vi "Numerical_Calculation.vi"(11 "Nums":sgl[][](array[numeric]) format="%#.2g") -> (3 "Calculation":sgl[][](array[numeric]) format="%#.2g")   [LabVIEW 2019]
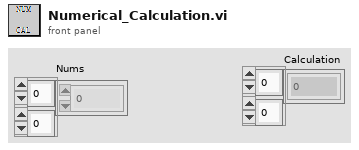
[diagram p1: front panel]
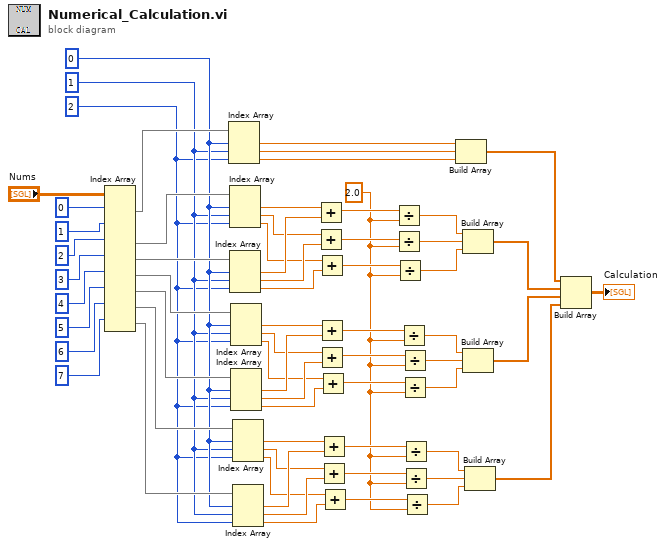
[diagram p0: block diagram]
diagram:
  w18 = sgl 2.0
  w28 = 2
  w29 = 1
  w30 = 0
  n1 = Index Array(array="Nums", index (row) #1=0 ("索引 (行)"), index (row) #2=1 ("索引 (行)"), index (row) #3=2 ("索引 (行)"), index (row) #4=3 ("索引 (行)"), index (row) #5=4 ("索引 (行)"), index (row) #6=5 ("索引 (行)"), index (row) #7=6 ("索引 (行)"), index (row) #8=7 ("索引 (行)")) -> (element #1=w55:sgl[], element #3=w36:sgl[], element #4=w35:sgl[], element #5=w34:sgl[], element #6=w33:sgl[], element #7=w32:sgl[], element #8=w31:sgl[])  [unwired: 8 in, 1 out]
  n2 = Index Array(array=w55, index #1=w30, index #2=w29, index #3=w28) -> (element #1=w4:sgl, element #2=w3:sgl, element #3=w2:sgl)
  n3 = Index Array(array=w36, index #1=w30, index #2=w29, index #3=w28) -> (element #1=w54:sgl, element #2=w52:sgl, element #3=w50:sgl)
  n4 = Index Array(array=w35, index #1=w30, index #2=w29, index #3=w28) -> (element #1=w53:sgl, element #2=w51:sgl, element #3=w49:sgl)
  n5 = Index Array(array=w34, index #1=w30, index #2=w29, index #3=w28) -> (element #1=w48:sgl, element #2=w46:sgl, element #3=w44:sgl)
  n6 = Index Array(array=w33, index #1=w30, index #2=w29, index #3=w28) -> (element #1=w47:sgl, element #2=w45:sgl, element #3=w43:sgl)
  n7 = Index Array(array=w32, index #1=w30, index #2=w29, index #3=w28) -> (element #1=w42:sgl, element #2=w40:sgl, element #3=w38:sgl)
  n8 = Index Array(array=w31, index #1=w30, index #2=w29, index #3=w28) -> (element #1=w41:sgl, element #2=w39:sgl, element #3=w37:sgl)
  n9 = Add(x=w54, y=w53) -> (x+y=w27:sgl)
  n10 = Add(x=w52, y=w51) -> (x+y=w26:sgl)
  n11 = Add(x=w50, y=w49) -> (x+y=w25:sgl)
  n12 = Add(x=w48, y=w47) -> (x+y=w24:sgl)
  n13 = Add(x=w46, y=w45) -> (x+y=w23:sgl)
  n14 = Add(x=w44, y=w43) -> (x+y=w22:sgl)
  n15 = Add(x=w42, y=w41) -> (x+y=w21:sgl)
  n16 = Add(x=w40, y=w39) -> (x+y=w20:sgl)
  n17 = Add(x=w38, y=w37) -> (x+y=w19:sgl)
  n18 = Divide(x=w27, y=w18) -> (x/y=w17:sgl)
  n19 = Divide(x=w26, y=w18) -> (x/y=w16:sgl)
  n20 = Divide(x=w25, y=w18) -> (x/y=w15:sgl)
  n21 = Divide(x=w24, y=w18) -> (x/y=w13:sgl)
  n22 = Divide(x=w23, y=w18) -> (x/y=w14:sgl)
  n23 = Divide(x=w22, y=w18) -> (x/y=w12:sgl)
  n24 = Divide(x=w21, y=w18) -> (x/y=w10:sgl)
  n25 = Divide(x=w20, y=w18) -> (x/y=w11:sgl)
  n26 = Divide(x=w19, y=w18) -> (x/y=w9:sgl)
  n27 = Build Array(w4, w3, w2) -> (w1:sgl[])
  n28 = Build Array(w17, w16, w15) -> (w8:sgl[])
  n29 = Build Array(w13, w14, w12) -> (w7:sgl[])
  n30 = Build Array(w10, w11, w9) -> (w6:sgl[])
  n31 = Build Array(w1, w8, w7, w6) -> (→"Calculation":sgl[][])
